vi "New Report Page.vi"(0 "report in":refnum<class "NI_report.lvclass">, 9 "MS Office parameters":T1, 11 "error in (no error)":errorcluster) -> (4 "report out":refnum<class "NI_report.lvclass">, 15 "error out":errorcluster)   [LabVIEW 2020, in "NI_report.lvclass"]
doc: "Creates a page break within the report."
uses:
  <vilib>/Utility/NIReport.llb/NI_report.lvclass
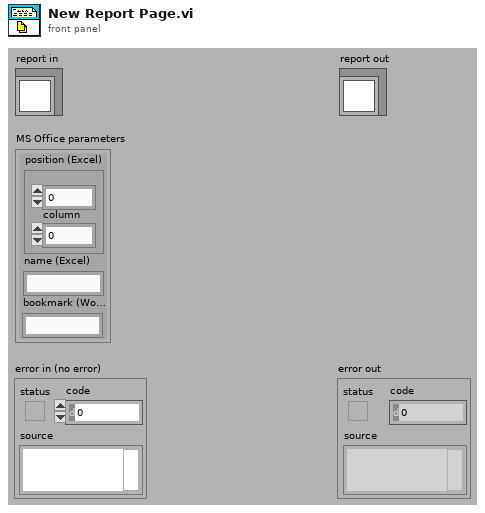
[diagram p1: front panel]
types:
  T1 = cluster{"position (Excel)":cluster{"row":i32, "column":i32}, "name (Excel) ":string, "bookmark (Word)":string}
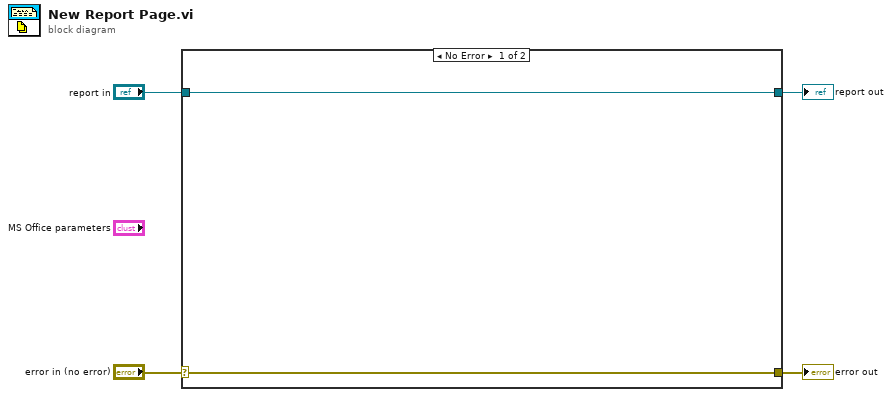
[diagram p0: block diagram]
diagram:
  n1 = case shown="No Error" "error in (no error)" {
    selector: "error in (no error)" -> [w5 w8]
    tunnel: [w5 w8] -> w3
    tunnel: [w6 w7] -> w1
    tunnel: "report in" -> [w6 w7]
    frame No Error {
    }
    frame Error {
    }
  }
  "error out" <- w3
  "report out" <- w1
